vi "Configure Current Of Sequence.vi"(8 "error in (no error)":errorcluster, 9 "Value(0)":dbl min=0.0, 10 "SEQ STEP(1)":u8=1 min=1 max=10 step=1, 11 "VISA resource name":refnum<visa-resource-name>) -> (0 "error out":errorcluster, 3 "VISA resource name out":refnum<visa-resource-name>)   [LabVIEW 2020, in "IT6500.lvlib"]
doc: "This command is used to edit the list sequence step current values.\n\n<b>SEQ STEP(1)</b>\nParameter 1 is the step to be edited (1 ~ 10). \n<b>Value (0)</b>\nParameter 2 is the current value (MIN ~ MAX).\nuint:A"
uses:
  IT6500.lvlib
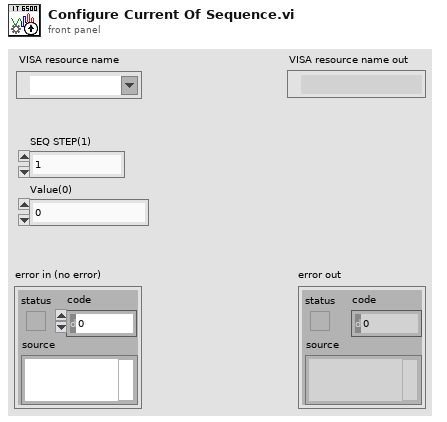
[diagram p1: front panel]
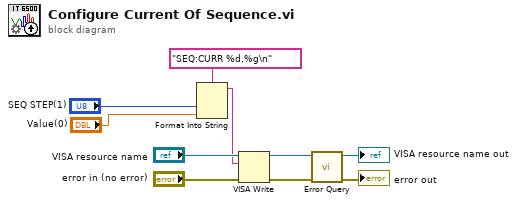
[diagram p0: block diagram]
diagram:
  n1 = Format Into String(format string="SEQ:CURR %d,%g\n", "SEQ STEP(1)", "Value(0)") -> (resulting string=w4:string)  [unwired: 2 in, 1 out]
  n2 = VISA Write(VISA resource name="VISA resource name", write buffer=w4, error in (no error)="error in (no error)") -> (VISA resource name out=w7:refnum<visa-resource-name>, error out=w8:errorcluster)  [unwired: 1 out]
  n3 = call "Error Query.vi"("error in (no error)"=w8, "VISA resource name"=w7) -> ("error out"=→"error out":errorcluster, "VISA resource name out"=→"VISA resource name out":refnum<visa-resource-name>)  [unwired: 6 in, 2 out]
